vi "System.Processes.vi"(7 "Partial Match":bool, 8 "error in":errorcluster, 9 "Process Names":string[](array[string]), 10 "Kill":bool, 11 "Process Name":string) -> (0 "error out":errorcluster, 1 "Was Killed":bool, 2 "Is Running":bool, 3 "Processes":string[](array[string]))   [LabVIEW 2019]
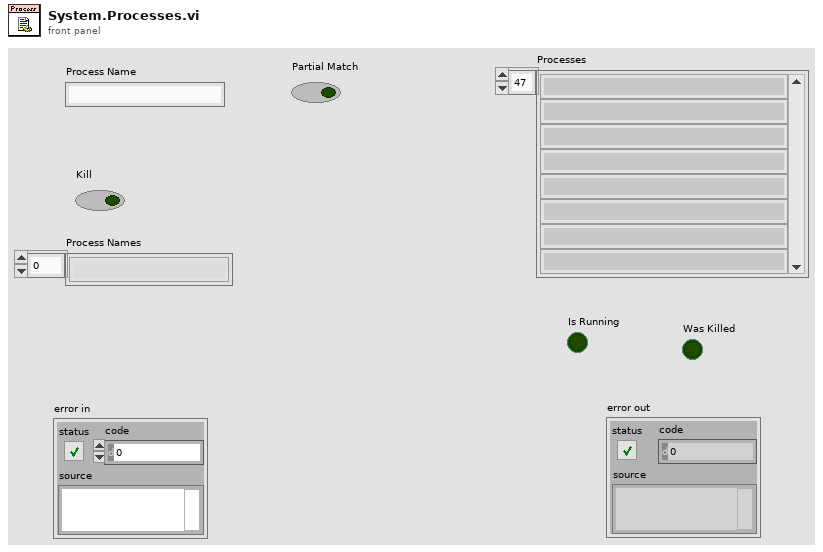
[diagram p1: front panel]
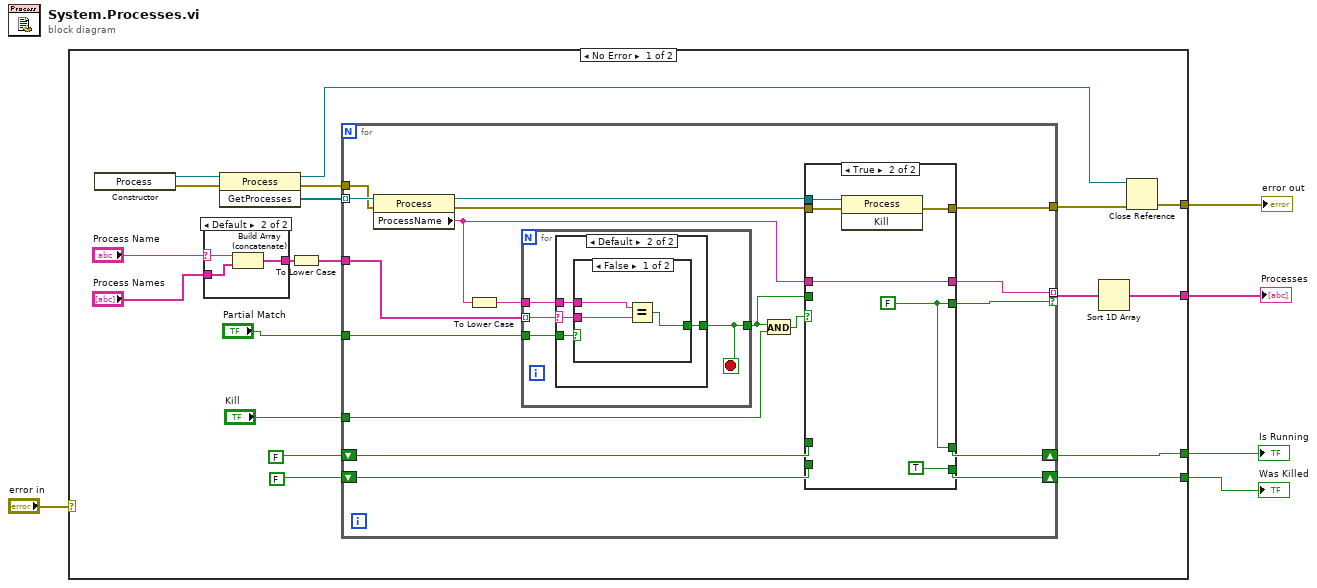
[diagram p0: block diagram]
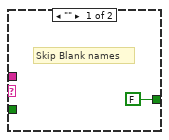
[diagram p3: hidden frame]
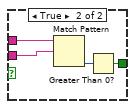
[diagram p4: hidden frame]
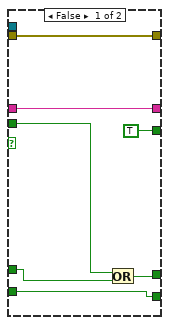
[diagram p5: hidden frame]
diagram:
  n1 = case shown="No Error" "error in" {
    selector: "error in" -> [_ w76]
    tunnel: [w17 w76] -> w5
    tunnel: [w13 _] -> w4
    tunnel: [w15 _] -> w3
    tunnel: [w6 _] -> w1
    frame No Error {
      n2 = constructor class="Process"() -> (reference out=w24:refnum<k24>, error out=w23:errorcluster)  [unwired: 3 in, 1 out]
      n3 = case shown="Default" "Process Name" {
        selector: "Process Name" -> [_ w28]
        tunnel: "Process Names" -> [w25 w27]
        tunnel: [w25 w26] -> w9
        frame "" {
        }
        frame Default {
          n4 = Build Array (concatenate)(w28, w27) -> (w26:string[])
        }
      }
      n5 = invoke class="Process" method="GetProcesses"(reference=w24, error in=w23) -> (reference out=w18:refnum<k24>, error out=w21:errorcluster, "GetProcesses"=w22:refnum<k24>[])  [unwired: 1 in]
      n6 = To Lower Case(string=w9) -> (all lower case string=w8:string[])
      n7 = for {
        tunnel: w22 -> [w46] mode=indexing
        tunnel: w21 -> [w43]
        tunnel: "Kill" -> [w42]
        tunnel: [w40] -> w14 mode=indexing if=w38
        tunnel: [w39] -> w19
        shift-right: [w37] -> w15
        shift-left: FALSE -> [w36]
        tunnel: "Partial Match" -> [w32]
        tunnel: w8 -> [w31]
        shift-right: [w29] -> w6
        shift-left: FALSE -> [w30]
        n8 = property class="Process"(reference=w46, error in=w43) -> (reference out=w45:refnum<k24>, error out=w44:errorcluster, "ProcessName"=w35:string)
        n9 = To Lower Case(string=w35) -> (all lower case string=w34:string)
        n10 = for {
          tunnel: w34 -> [w50]
          tunnel: w31 -> [w49] mode=indexing
          tunnel: w32 -> [w48]
          tunnel: [w47] -> w33
          stop <- w47 stop-if-true
          n11 = case shown="Default" w49 {
            selector: w49 -> [_ w54]
            tunnel: w50 -> [_ w55]
            tunnel: w48 -> [_ w53]
            tunnel: [FALSE w52] -> w47
            frame "" {
              # "Skip Blank names"
            }
            frame Default {
              n12 = case shown="False" w53 {
                tunnel: w55 -> [w58 w62]
                tunnel: w54 -> [w57 w61]
                tunnel: [w56 w59] -> w52
                frame False {
                  n13 = Equal?(x=w58, y=w57) -> (x = y?=w56:bool)
                }
                frame True {
                  n14 = Match Pattern(string=w62, regular expression=w61) -> (offset past match=w60:i32)  [unwired: 1 in, 3 out]
                  n15 = Greater Than 0?(x=w60) -> (x > 0?=w59:bool)
                }
              }
            }
          }
        }
        n16 = And(x=w33, y=w42) -> (x .and. y?=w41:bool)
        n17 = case shown="True" w41 {
          tunnel: w45 -> [_ w75]
          tunnel: w44 -> [w67 w74]
          tunnel: w35 -> [w68 w73]
          tunnel: [w68 w73] -> w40
          tunnel: [w67 w72] -> w39
          tunnel: [TRUE w71] -> w38
          tunnel: [w66 w71] -> w37
          tunnel: w33 -> [w65 _]
          tunnel: w36 -> [w64 _]
          tunnel: [w63 TRUE] -> w29
          tunnel: w30 -> [w63 _]
          frame False {
            n18 = Or(x=w65, y=w64) -> (x .or. y?=w66:bool)
          }
          frame True {
            w71 = FALSE
            n19 = invoke class="Process" method="Kill"(reference=w75, error in=w74) -> (error out=w72:errorcluster)  [unwired: 1 in, 2 out]
          }
        }
      }
      n20 = Sort 1D Array(array=w14) -> (sorted array=w13:string[])
      n21 = Close Reference(reference=w18, error in (no error)=w19) -> (error out=w17:errorcluster)
    }
    frame Error {
    }
  }
  "Is Running" <- w3
  "error out" <- w5
  "Processes" <- w4
  "Was Killed" <- w1
